vi "Fast Get Item Children FuncGlobal.vi"(5 "Action":enum16{"Open or Add", "Close Ref"}(ring), 8 "error in (no error)":errorcluster, 11 "Item Ref in":T1 format="%.0x") -> (0 "error out":errorcluster, 2 "Child Refs":T1[](array[typedef]) format="%.0x", 3 "Item Ref out":T1 format="%.0x", 4 "Found":bool)   [LabVIEW 2011]
doc: "Returns a list of references to all child items of the specified item. This list can include subsections and channels."
uses:
  <vilib>/NI Veristand/Custom Device API/Custom Device Item Ref.ctl
  <vilib>/NI Veristand/Custom Device API/Custom Device API.lvlib
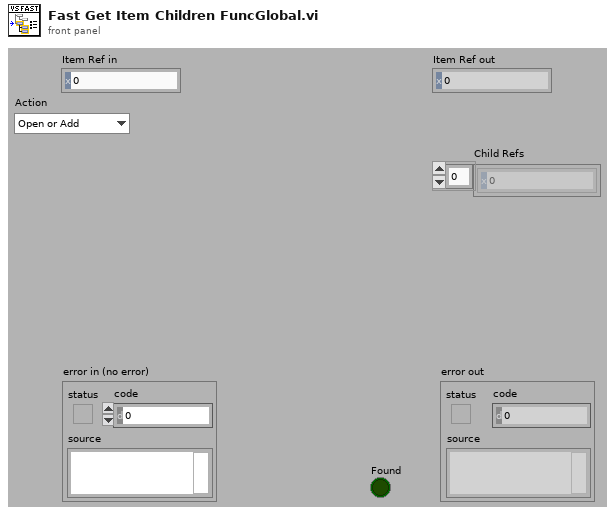
[diagram p1: front panel]
types:
  T1 = typedef "Custom Device API.lvlib/Custom Device Item Ref.ctl" = u64
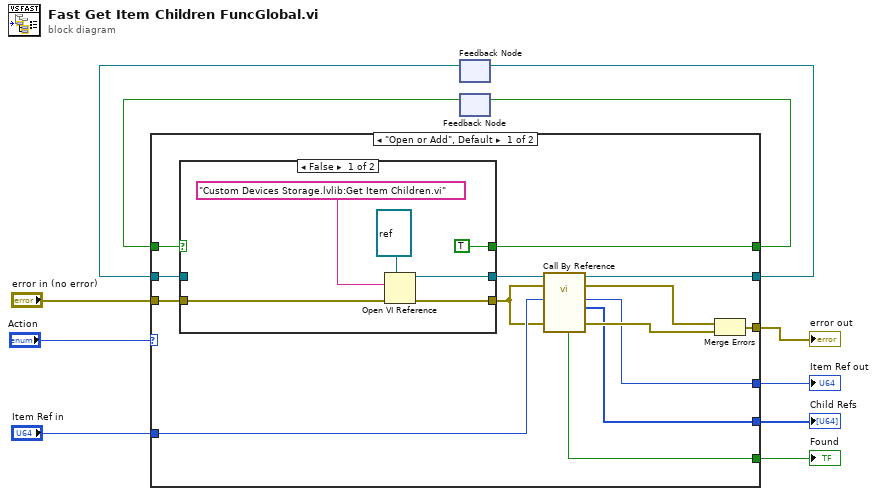
[diagram p0: block diagram]
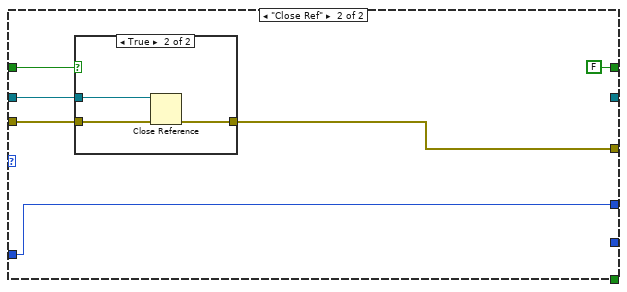
[diagram p3: hidden frame]
diagram:
  n1 = feedback #1() -> (w2:refnum<vi>)  [unwired: 1 in]
  n2 = feedback #2() -> (w3:bool)  [unwired: 1 in]
  n3 = case shown="\"Open or Add\", Default" "Action" {
    tunnel: [w24 w37] -> w11
    tunnel: "Item Ref in" -> [w23 w35]
    tunnel: [w22 w35] -> w9
    tunnel: [w21 _] -> w8
    tunnel: [w20 _] -> w7
    tunnel: "error in (no error)" -> [w19 w38]
    tunnel: [w15 _] -> w5
    tunnel: [w14 FALSE] -> w4
    tunnel: w3 -> [w12 w40]
    tunnel: w2 -> [w13 w39]
    frame "Open or Add", Default {
      n4 = case shown="False" w12 {
        selector: w12 -> [_ w32]
        tunnel: w19 -> [w29 w34]
        tunnel: [w28 w34] -> w18
        tunnel: [w27 w33] -> w17
        tunnel: [TRUE w32] -> w14
        tunnel: w13 -> [_ w33]
        frame False {
          n5 = Open VI Reference(type specifier VI Refnum (for type only)=refnum<vi> refnum, vi path="Custom Devices Storage.lvlib:Get Item Children.vi", error in (no error)=w29) -> (vi reference=w27:refnum<vi>, error out=w28:errorcluster)  [unwired: 3 out]
        }
        frame True {
        }
      }
      n6 = call-by-ref "?"(reference=w17, error in=w18, 8:"error in (no error)"=w18, "Item Ref in"=w23) -> (reference out=w15:refnum<vi>, error out=w16:errorcluster, 0:"error out"=w25:errorcluster, "Child Refs"=w21:T1[], "Item Ref out"=w22:T1, "Found"=w20:bool)  [unwired: 6 in]
      n7 = Merge Errors(w16, w25) -> (w24:errorcluster)
    }
    frame "Close Ref" {
      n8 = case shown="True" w40 {
        tunnel: w39 -> [_ w44]
        tunnel: w38 -> [w41 w43]
        tunnel: [w41 w42] -> w37
        frame False {
        }
        frame True {
          n9 = Close Reference(reference=w44, error in (no error)=w43) -> (error out=w42:errorcluster)
        }
      }
    }
  }
  "Item Ref out" <- w9
  "error out" <- w11
  "Found" <- w7
  "Child Refs" <- w8
  n10 = feedback-in #1(w5) -> ()
  n11 = feedback-in #2(w4) -> ()
